vi "Set Audio Device Volume.vi"(8 "error in (no error)":errorcluster, 10 "Volume":sgl, 11 "Audio Device Refnum In":T1) -> (0 "error out":errorcluster, 3 "Audio Device Refnum Out":T1)   [LabVIEW 2020, in "G-Audio.lvlib"]
doc: "Set the audio device volume. Applies to playback and capture devices.\n\n<b>Volume</b> should be between 0 and 1 inclusive. A volume less than 0 will result in an error. A volume greater than 1 won't generate an error, but may cause clipping."
uses:
  G-Audio.lvlib
  lib/g_audio_32.dll
  Controls/Audio Device Refnum.ctl
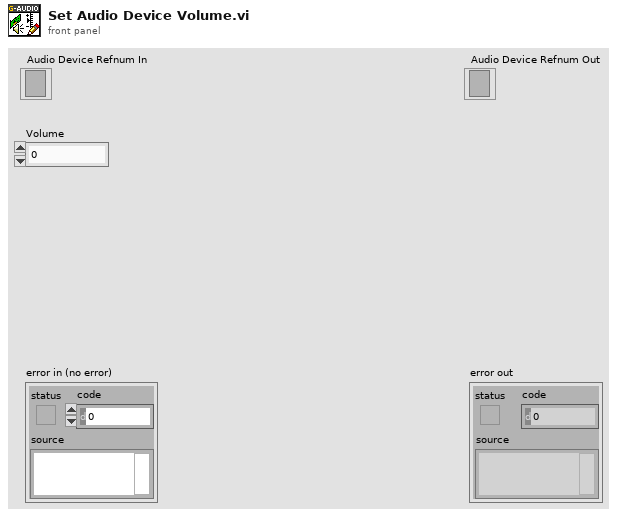
[diagram p1: front panel]
types:
  T1 = typedef "G-Audio.lvlib/Audio Device Refnum.ctl" = refnum<file>
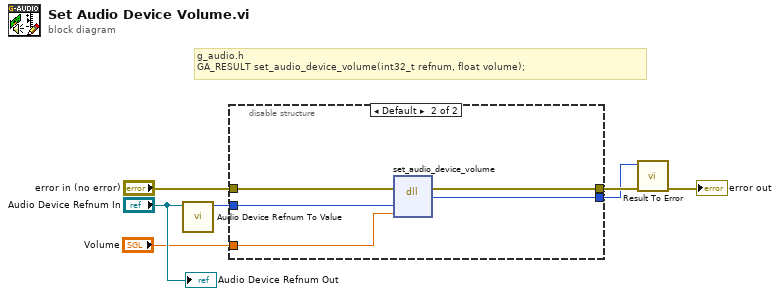
[diagram p0: block diagram]
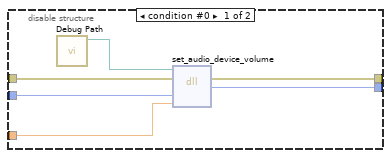
[diagram p2: hidden frame]
diagram:
  # "g_audio.h\nGA_RESULT set_audio_device_volume(int32_t refnum, float volume);"
  n1 = call "Audio Device Refnum To Value.vi"("Audio Device Refnum"="Audio Device Refnum In") -> ("Refnum Value"=w5:i32)  [unwired: 10 in]
  n2 = disable-structure shown="Default" {
    disable-tunnel: [w12 w18] -> w7
    disable-tunnel: [w11 w17] -> w6
    disable-tunnel: w5 -> [w10 w16]
    disable-tunnel: "error in (no error)" -> [w9 w15]
    disable-tunnel: "Volume" -> [w8 w14]
    frame condition #0 {
      n3 = call "Debug Path.vi"() -> ("Debug Path"=w13:path)  [unwired: 11 in]
      n4 = dll-call lib="?" fn="set_audio_device_volume"(path in=w13, error in=w9, "refnum"=w10, "volume"=w8) -> (error out=w12:errorcluster, "result"=w11:i32)  [unwired: 3 in, 1 out]
    }
    frame condition #1 (active) {
      n5 = dll-call lib="C:/github/dataflowg/g-audio/src/LabVIEW/G-Audio/lib/g_audio_*.*" fn="set_audio_device_volume"(error in=w15, "refnum"=w16, "volume"=w14) -> (error out=w18:errorcluster, "result"=w17:i32)  [unwired: 4 in, 1 out]
    }
  }
  n6 = call "Result To Error.vi"("error in (no error)"=w7, "Result Code"=w6) -> ("error out"=→"error out":errorcluster)  [unwired: 9 in]
  "Audio Device Refnum Out" <- "Audio Device Refnum In"
